vi "PatternMatch_Setting_UI.vi"(0 "Vision_Image In":T4(plugin-control), 1 "Coord?":bool, 3 "Type":string, 5 "List ROI Ref":refnum<vi>, 7 "AlgIn":T2, 9 "ProjectName":string="CDF", 11 "error in (no error)":errorcluster, 12 "ParameterIn":string, 14 "RootPath":path) -> (6 "ParameerOut":string, 10 "Cancel?":bool, 15 "error out":errorcluster)   [LabVIEW 2019]
uses:
  Controls/Parttern Match/Analysis_PatternMatch_Result.ctl
  Controls/V_Analysis_Type.ctl
  Controls/_UI Command Cluster/Pattern Match_UI Command.ctl
  <vilib>/Utility/miscctls.llb/LVPointTypeDef.ctl
  Controls/Analysis_Setting.ctl
  Controls/Parttern Match/Analysis_PatternMatch_Parameter.ctl
  <vilib>/vision/Image Controls.llb/IMAQ Image.ctl
  11e1650d-9a27-4c98-b785-94bb4e51b252.vi
  fe4c8c9f-3b30-4d10-b5c7-71603a67618a.vi
  c6f29bbc-09ff-4359-9596-1a03bc10ebeb.vi
  a50e33b9-da3b-4096-9a32-63f0ae2ad806.vi
  7765c890-54c4-40a3-a063-9b2138e01ba1.vi
  ff688e6c-f413-41b3-9d93-3794729c7324.vi
  <vilib>/JDP Science/JSONtext/JSON text to Variant.vi
  <vilib>/JDP Science/JSONtext/Variant to JSON Text.vi
  <vilib>/vision/NI_Vision_Development_Module.lvlib
  <vilib>/userdefined/High Color/IMAQdx.ctl
panel:
  out "ListROI":T1
  out "Algout":T2=enum."G_PatternMatching"
  out "Matches (real-world)":T3(array[cluster]) {"Bounding Box"."y" format="%.2f"; "Bounding Box"."x" format="%.2f"; "Score" format="%.2f"; "Scale" format="%.2f"; "Angle" format="%.2f"; "Position"."y" format="%.2f"; "Position"."x" format="%.2f"}
  in  "SetROI":bool
  out "ROI":T1
  out "Template Image":T4(plugin-control)
  in  "Cancel":bool
  in  "Done":bool
  in  "PatternMatchTab":T5(tab)
  in  "Y Position Offset":i32
  in  "X Position Offset":i32
  in  "Match Parameters":T6={"Number of Matches Requested"=1, "Minimum Match Score"=750.0, "Angle Ranges"=[]} {"Angle Ranges"."End Angle" min=-360 max=360; "Angle Ranges"."Start Angle" min=-360 max=360; "Minimum Match Score" min=0 max=1000; "Number of Matches Requested" min=1 max=9999}
  in  "Algorithm":i32(ring)=1 items=["All", "Low Discrepancy Sampling", "Grayscale Value Pyramid", "Gradients Pyramid"]
  in  "Advanced Options":cluster{"Item":u16, "Value":dbl}[](array[cluster])=[{"Item"=1, "Value"=1.0}, {"Item"=103, "Value"=1.0}] {"Item" items=["LD Sampling - Minimum Constrast"=0, "LD Sampling - Enable Subpixel Accuracy"=1, "LD Sampling - Search Strategy"=2, "LD Sampling - Subpixel Iterations"=3, "LD Sampling - Subpixel Tolerance"=4, "LD Sampling - Initial Match List Length"=5, "LD Sampling - Match List Reduction Factor"=6, "LD Sampling - Initial Step Size"=7, "LD Sampling - Intermediate Angular Accuracy"=8, "-"=9, "Pyramid - Max Pyramid Level"=100, "Pyramid - Minimum Contrast"=102, "Pyramid - Enable Subpixel Accuracy"=103, "Pyramid - Subpixel Iterations"=104, "Pyramid - Subpixel Tolerance"=105, "Pyramid - Initial Match List Length"=106, "Pyramid - Match List Reduction Factor"=107, "Pyramid - Intermediate Angular Accuracy"=108, "Pyramid - Process Border Matches"=109, "Pyramid - Min Match Separation Distance"=111, "Pyramid - Min Match Separation Angle"=112, "Pyramid - Max Match Overlap"=113, "Pyramid - Max Cache in MB"=114, "Pyramid - Clear Cache"=115]}
  out "Matches":T7[](array[typedef]) {"Bounding Box"."y" format="%.2f"; "Bounding Box"."x" format="%.2f"; "Score" format="%.2f"; "Scale" format="%.2g"; "Angle" format="%.2f"; "Position"."y" format="%.2f"; "Position"."x" format="%.2f"}
  in  "Vision_Image":T4(plugin-control)
  in  "Run Algorithm":bool
  in  "SetTemplate":bool
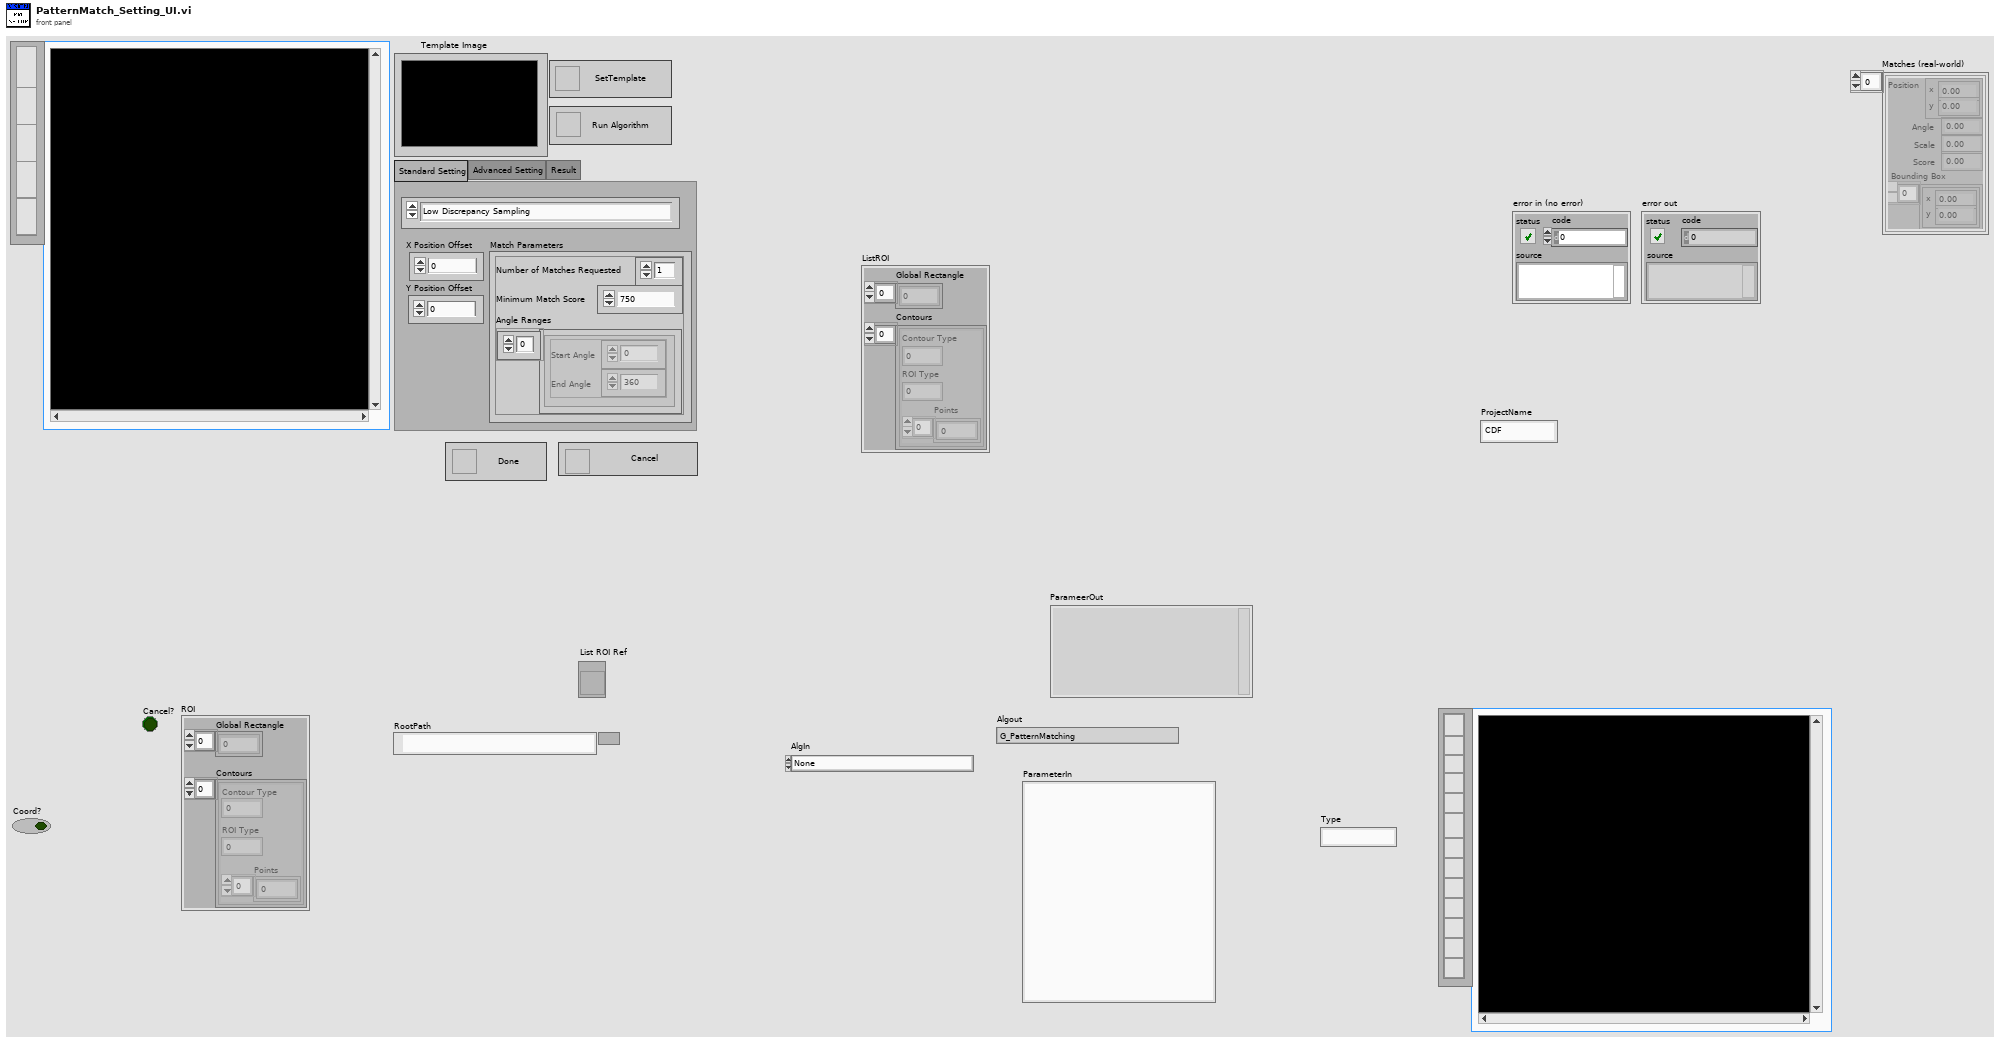
[diagram p1: front panel]
types:
  T1 = cluster{"Global Rectangle":i32[], "Contours":cluster{"Contour Type":u32, "ROI Type":u32, "Points":i32[]}[]}
  T2 = typedef "V_Analysis_Type.ctl" = enum16{"None", "C_Color Pattern Matching", "G_PatternMatching", "G_ShapeDectect", "G_GeometricMatch", "B_Area Check"}
  T3 = cluster{"Position":cluster{"x":sgl, "y":sgl}, "Angle":sgl, "Scale":sgl, "Score":sgl, "Bounding Box":cluster{"x":sgl, "y":sgl}[]}[]
  T4 = typedef "IMAQ Image.ctl" = refnum<image>
  T5 = enum32{"Standard Setting", "Advanced Setting", "Result"}
  T6 = cluster{"Number of Matches Requested":i32, "Minimum Match Score":sgl, "Angle Ranges":cluster{"Start Angle":sgl, "End Angle":sgl}[]}
  T7 = typedef "Analysis_PatternMatch_Result.ctl" = cluster{"Position":cluster{"x":sgl, "y":sgl}, "Angle":sgl, "Scale":sgl, "Score":sgl, "Bounding Box":cluster{"x":sgl, "y":sgl}[]}
  T8 = typedef "Image Type" = u32
  T9 = typedef "Pattern Match_UI Command.ctl" = enum16{"Init", "Done", "Cancel", "RunAlgorithm", "SetTemplate", "SetROI", "ClearOverlay", "Load Template", "Draw Overlay", "Offset", "Draw Curve"}
  T10 = typedef "LVPointTypeDef.ctl" = cluster{"Horizontal":i16, "Vertical":i16}
  T11 = typedef "IMAQdx.ctl" = refnum<k21>
  T12 = typedef "Analysis_Setting.ctl" = cluster{"PreProcess":T2, "Parameter":string}
  T13 = enum8{"Enabled", "Disabled", "Disabled and Grayed Out"}
  T14 = typedef "ROI Descriptor" = cluster{"Global Rectangle":i32[], "Contours":cluster{"ID":enum32{"External", "Internal"}, "Type":u32, "Coordinates":i32[]}[]}
  T15 = cluster{"Algorithm":i32, "Match Parameters":cluster{"Number of Matches Requested":i32, "Minimum Match Score":sgl, "Angle Ranges":cluster{"Start Angle":sgl, "End Angle":sgl}[]}, "ROI Descriptor":T14, "Advanced Options":cluster{"Item":u16, "Value":dbl}[], "Template path":string}
  T16 = typedef "Analysis_PatternMatch_Parameter.ctl" = cluster{"Algorithm":i32, "Match Parameters":cluster{"Number of Matches Requested":i32, "Minimum Match Score":sgl, "Angle Ranges":cluster{"Start Angle":sgl, "End Angle":sgl}[]}, "ROI Descriptor":T14, "Advanced Options":cluster{"Item":u16, "Value":dbl}[], "Template path":string, "XOffset":i32, "YOffset":i32}
  T17 = cluster{"Algorithm":i32, "Match Parameters":cluster{"Number of Matches Requested":i32, "Minimum Match Score":sgl, "Angle Ranges":cluster{"Start Angle":sgl, "End Angle":sgl}[]}, "ROI":cluster{"Global Rectangle":i32[], "Contours":cluster{"Contour Type":u32, "ROI Type":u32, "Points":i32[]}[]}, "Advanced Options":cluster{"Item":u16, "Value":dbl}[], string, i32, i32}
  T18 = cluster{"Contour Type":u32, "ROI Type":u32, "Points":i32[]}[]
  T19 = enum16{"Init", "Done", "Cancel", "RunAlgorithm", "SetTemplate", "SetROI", "ClearOverlay"}
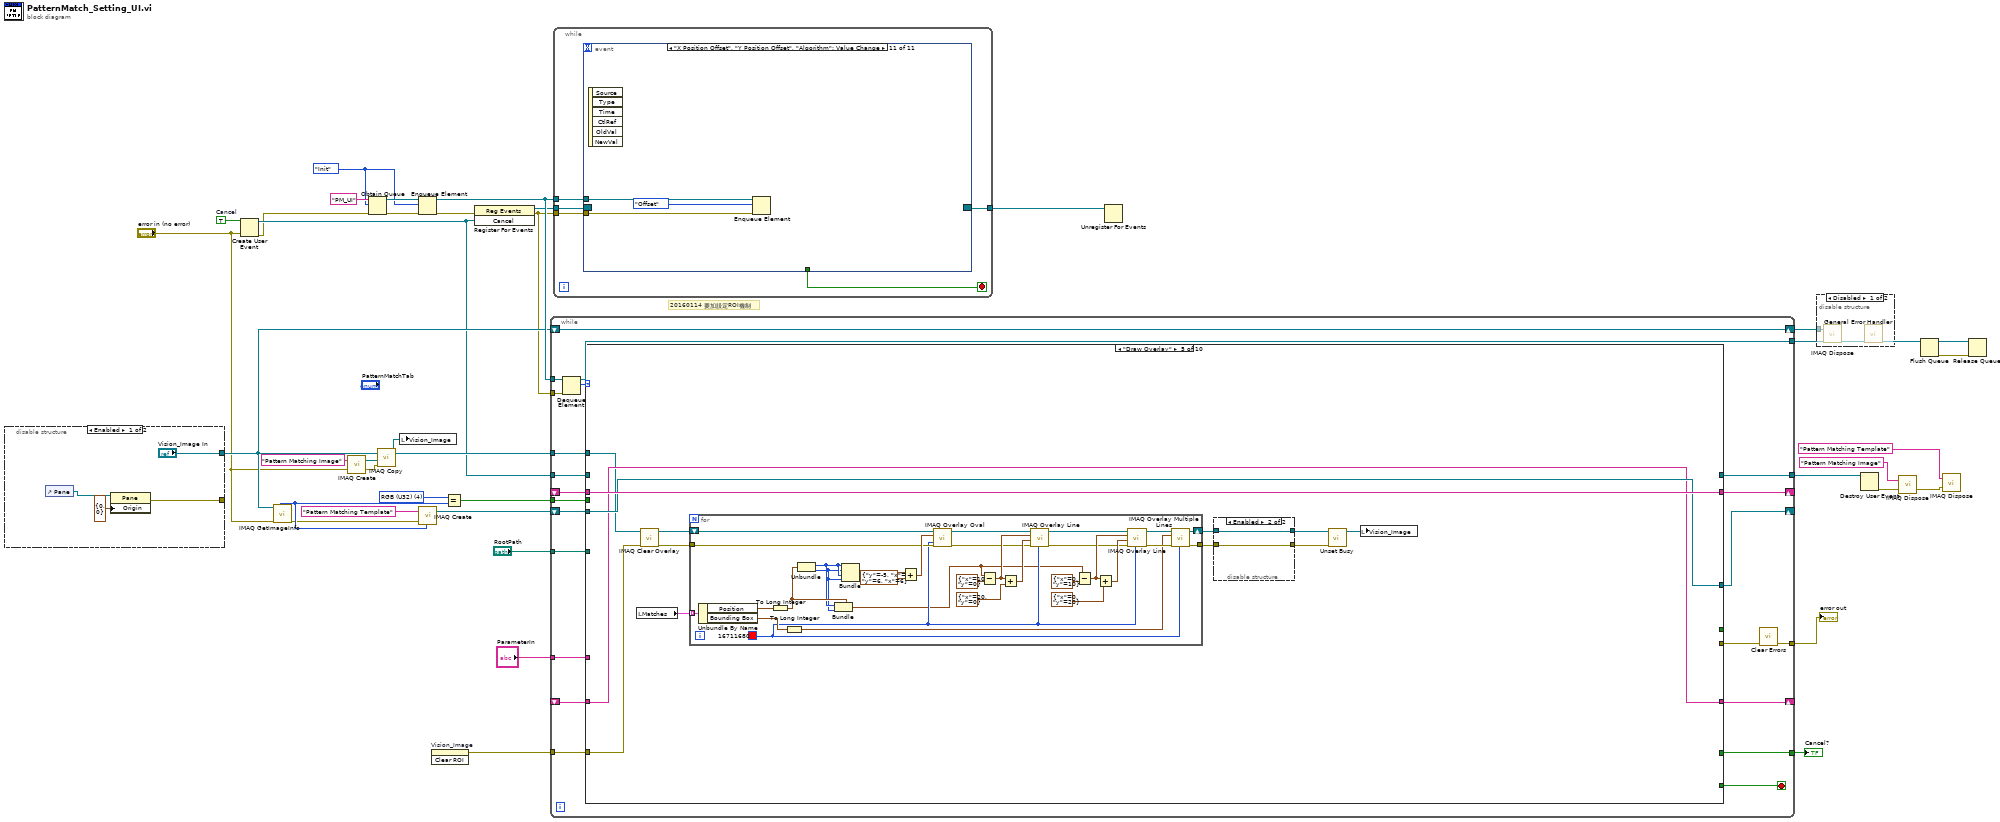
[diagram p0: block diagram]
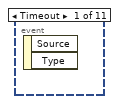
[diagram p2: hidden frame]
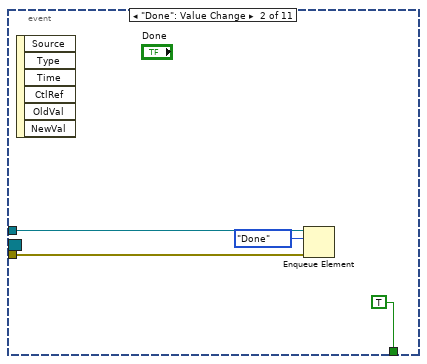
[diagram p3: hidden frame]
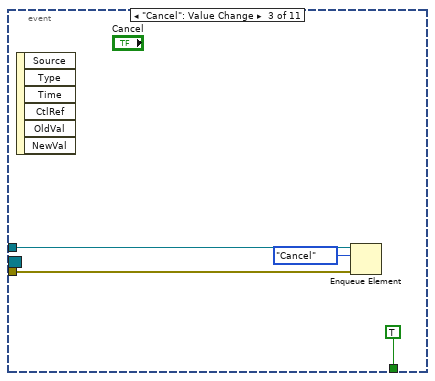
[diagram p4: hidden frame]
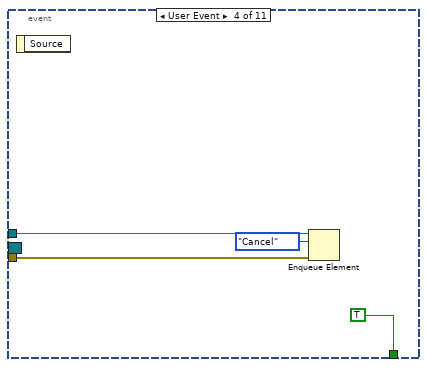
[diagram p5: hidden frame]
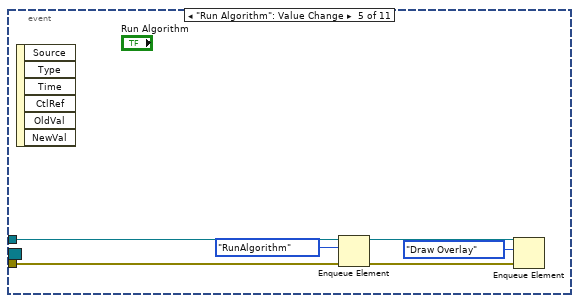
[diagram p6: hidden frame]
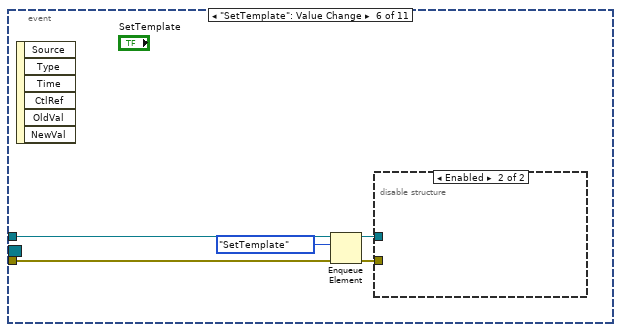
[diagram p7: hidden frame]
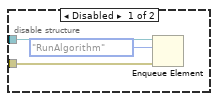
[diagram p8: hidden frame]
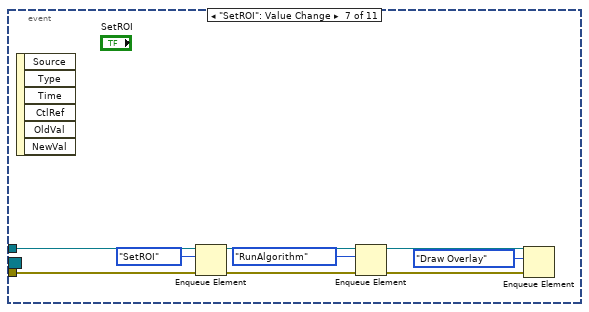
[diagram p9: hidden frame]
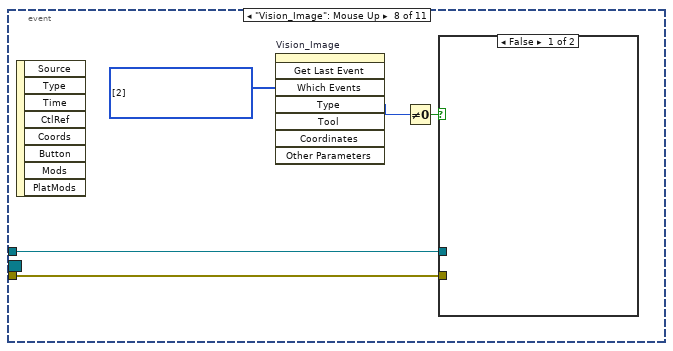
[diagram p10: hidden frame]
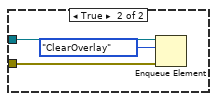
[diagram p11: hidden frame]
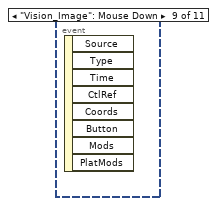
[diagram p12: hidden frame]
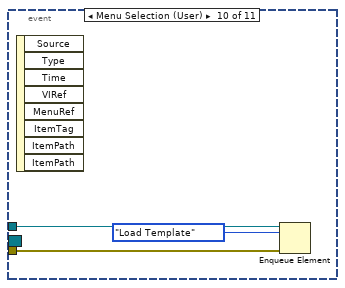
[diagram p13: hidden frame]
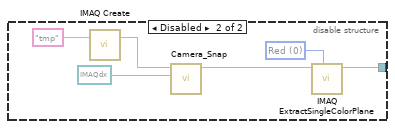
[diagram p14: hidden frame]
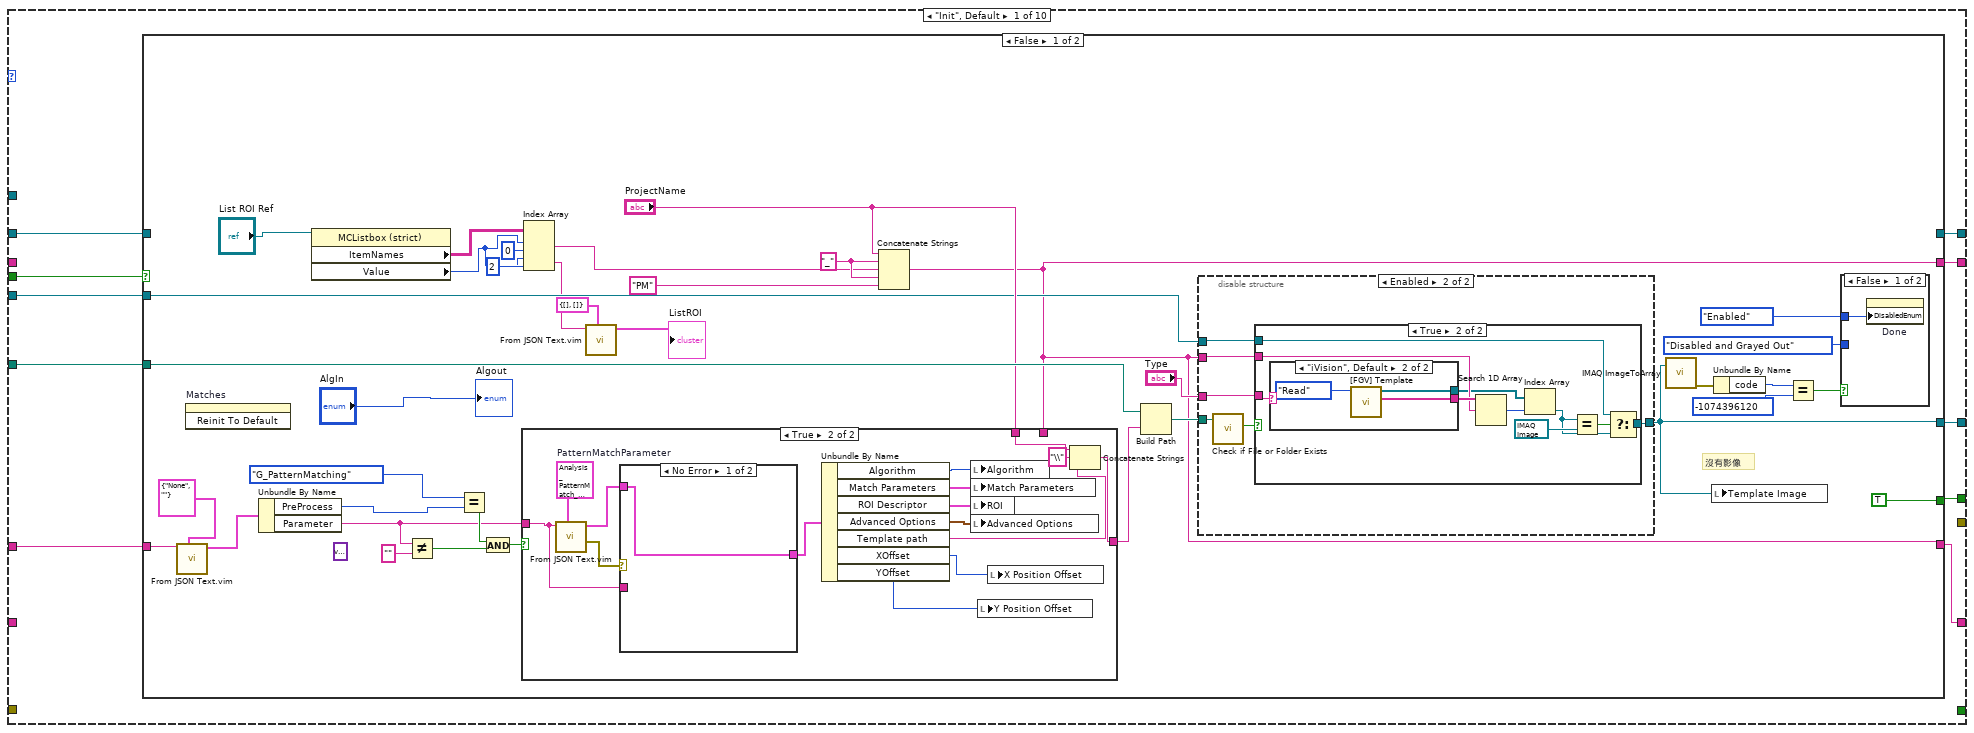
[diagram p16: hidden frame]
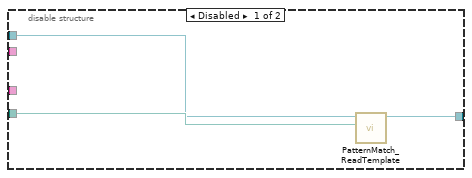
[diagram p17: hidden frame]
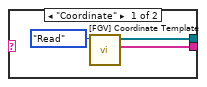
[diagram p19: hidden frame]
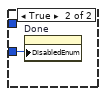
[diagram p20: hidden frame]
diagram:
  w18 = TRUE  # Cancel
  w20 = T8 4 items=["Grayscale (U8)", "Grayscale (I16)", "Grayscale (SGL)", "Complex (CSG)", "RGB (U32)", "HSL (U32)", "RGB (U64)", "Grayscale (U16)"] ("x")
  w19 = Pattern_Match_UI_Command."Init"
  # "20160114 要加設定ROI機制"
  n1 = disable-structure shown="Enabled" {
    disable-tunnel: ["Vision_Image In" w44] -> w24
    disable-tunnel: [w39 _] -> _
    frame Enabled {
      n2 = control-ref of="Pane"() -> (w41:refnum<vi>)
      n3 = property class="Pane"(reference=w41, "Origin"=T10 {"Horizontal"=0, "Vertical"=0}) -> (error out=w39:errorcluster)  [unwired: 1 in, 1 out]
    }
    frame Disabled {
      w43 = 0 items=["Red", "Green", "Blue", "Hue", "Saturation", "Luminance", "Value", "Intensity"] ("Color Plane")
      n4 = call "IMAQ Create"("Image Name"="tmp") -> ("New Image"=w46:T4)  [unwired: 4 in, 1 out]
      n5 = call "Camera_Snap.vi"("Camera Session In"=T11 refnum, "Image In"=w46) -> ("New Image"=w45:T4)  [unwired: 8 in, 1 out]
      n6 = call "IMAQ ExtractSingleColorPlane"("Color Plane"=w43, "Image Src"=w45) -> ("Image Dst Out"=w44:T4)  [unwired: 2 in, 7 out]
    }
  }
  n7 = Create User Event(user event datatype=w18, error in="error in (no error)") -> (user event=w15:refnum<user-event>, error out=w6:errorcluster)
  n8 = call "IMAQ GetImageInfo"("error in (no error)"="error in (no error)", "Image"=w24) -> ("error out"=w4:errorcluster, "Image Type"=w21:T8)  [unwired: 2 in, 6 out]
  n9 = call "IMAQ Create"("Image Name"="Pattern Matching Image", "error in (no error)"="error in (no error)") -> ("New Image"=w33:T4, "error out"=w5:errorcluster)  [unwired: 3 in]
  n10 = Obtain Queue(name (unnamed)="PM_UI", element data type=w19, error in (no error)=w6) -> (queue out=w30:refnum<queue>, error out=w29:errorcluster)  [unwired: 2 in, 1 out]
  n11 = call "IMAQ Copy"("error in (no error)"=w5, "Image Dst"=w33, "Image Src"=w24) -> ("Image Dst Out"=w32:T4)  [unwired: 3 in, 1 out]
  n12 = local write "Vision_Image"(w32) -> ()
  n13 = Enqueue Element(queue=w30, element=w19, error in (no error)=w29) -> (queue out=w26:refnum<queue>, error out=w12:errorcluster)  [unwired: 1 in, 1 out]
  n14 = call "IMAQ Create"("Image Name"="Pattern Matching Template", "Image Type"=w21, "error in (no error)"=w4) -> ("New Image"=w23:T4)  [unwired: 2 in, 1 out]
  n15 = invoke on="Vision_Image" class="ImageControl" method="Clear ROI"() -> (error out=w35:errorcluster)  [unwired: 3 in, 2 out]
  n16 = Equal?(x=w20, y=w21) -> (x = y?=w16:bool)
  n17 = register-events(error in=w12, w15) -> (reference out=w17:refnum<event-registration>, error out=w11:errorcluster)  [unwired: 1 in]
  n18 = while {
    shift-right: [w70] -> w38
    shift-left: w24 -> [w70]
    tunnel: [w66] -> w37
    tunnel: w35 -> [w52]
    tunnel: w32 -> [w69]
    tunnel: w26 -> [w64]
    tunnel: w11 -> [w62]
    tunnel: [w61] -> w25
    shift-right: [w60] -> _
    shift-left: _ -> [w59]
    shift-right: [w57] -> _
    shift-left: w23 -> [w68]
    shift-right: [w58] -> _
    shift-left: _ -> [w67]
    tunnel: "RootPath" -> [w56]
    tunnel: w16 -> [w55]
    tunnel: w15 -> [w54]
    tunnel: [w53] -> w14
    tunnel: [w51] -> w2
    tunnel: "ParameterIn" -> [w49]
    stop <- w65 stop-if-true
    n19 = Dequeue Element(queue=w64, error in (no error)=w62) -> (queue out=w61:refnum<queue>, element=w63:T9)  [unwired: 1 in, 2 out]
    n20 = case shown="\"Draw Overlay\"" w63 {
      tunnel: [_ TRUE w211 _ _ _ _ _ _ _] -> w65
      tunnel: w69 -> [_ w196 w210 _ w267 _ _ _ _ _]
      tunnel: w68 -> [w75 _ w209 w215 w269 w317 w395 w405 w419 w446]
      tunnel: [_ _ w211 _ _ _ _ _ _ _] -> w66
      tunnel: w67 -> [_ w193 w207 w213 w268 w318 w396 w406 w420 w430]
      tunnel: [w79 w195 w208 w220 w270 w319 w397 w407 w421 _] -> w60
      tunnel: w59 -> [_ w195 w208 w220 w270 w319 w397 w407 w421 _]
      tunnel: [w77 w193 w207 w213 w268 w318 w396 w406 w420 w430] -> w58
      tunnel: [w80 T4 refnum ("Template Out") T4 refnum ("Template Out") w215 w269 w314 w395 w405 w411 w432] -> w57
      tunnel: [w78 FALSE _ _ _ w316 _ _ _ _] -> _
      tunnel: w56 -> [w76 _ _ _ _ w315 _ _ w418 w431]
      tunnel: w55 -> [w74 _ _ _ _ _ _ _ _ _]
      tunnel: w54 -> [w73 w191 w205 _ _ _ _ _ _ _]
      tunnel: [w72 w191 w205 _ _ _ _ _ _ _] -> w53
      tunnel: w52 -> [_ _ _ _ w264 _ _ _ _ _]
      tunnel: [_ _ _ w212 _ _ _ _ _ _] -> w50
      tunnel: w49 -> [w71 _ _ _ _ _ _ _ _ _]
      frame "Init", Default {
        n21 = case shown="False" w74 {
          tunnel: [w105 _] -> w80
          tunnel: [w82 _] -> w79
          tunnel: [TRUE _] -> w78
          tunnel: [w82 _] -> w77
          tunnel: w76 -> [w116 _]
          tunnel: w75 -> [w106 _]
          tunnel: w73 -> [_ w182]
          tunnel: [_ w180] -> w72
          tunnel: w71 -> [w84 _]
          frame False {
            (unwired) variant
            w113 = "_" ("string")
            # "沒有影像"
            n22 = call "From JSON Text.vim"("Data Type and Default Value"=T12 {"PreProcess"=enum."None", "Parameter"=""} ("Analysis_Setting In"), "JSON"=w84) -> ("Data out"=w85:T12)  [unwired: 8 in, 1 out]
            n23 = invoke on="Matches" class="Arr (strict)" method="Reinit To Default"() -> ()  [unwired: 3 in, 3 out]
            n24 = Unbundle By Name(w85) -> ("PreProcess"=w83:T2, "Parameter"=w108:string)
            n25 = property class="MCListbox (strict)"(reference="List ROI Ref") -> ("ItemNames"=w92:string[][], "Value"=w91:i32)  [unwired: 1 in, 2 out]
            n26 = Not Equal?(x=w108, y="") -> (x != y?=w111:bool)
            n27 = Equal?(x=V_Analysis_Type."G_PatternMatching", y=w83) -> (x = y?=w112:bool)
            n28 = And(x=w112, y=w111) -> (x .and. y?=w109:bool)
            n29 = Index Array(array=w92, index (row) #1=w91, index (col) #1=0 ("disabled index (col)"), index (row) #2=w91, index (col) #2=2 ("disabled index (col)")) -> (element #1=w90:string, element #2=w88:string)
            n30 = call "From JSON Text.vim"("Data Type and Default Value"=T1 {"Global Rectangle"=[], "Contours"=[]} ("ROI"), "JSON"=w88) -> ("Data out"=→"ListROI":T1)  [unwired: 8 in, 1 out]
            n31 = Concatenate Strings("ProjectName", w113, w90, w113, "PM" ("string")) -> (w82:string)
            n32 = case shown="True" w109 {
              tunnel: [w146 w153] -> w81
              tunnel: "ProjectName" -> [w147 w156]
              tunnel: w108 -> [_ w159]
              tunnel: w82 -> [w148 _]
              frame False {
                n33 = invoke on="Y Position Offset" class="DigNum (strict)" method="Reinit To Default"() -> ()  [unwired: 3 in, 3 out]
                n34 = invoke on="X Position Offset" class="DigNum (strict)" method="Reinit To Default"() -> ()  [unwired: 3 in, 3 out]
                n35 = invoke on="Algorithm" class="Ring (strict)" method="Reinit To Default"() -> ()  [unwired: 3 in, 3 out]
                n36 = case shown="True" "Coord?" {
                  frame False {
                    n37 = invoke on="Match Parameters" class="Clust (strict)" method="Reinit To Default"() -> ()  [unwired: 3 in, 3 out]
                  }
                  frame True {
                    n38 = local write "Match Parameters"(T6 {"Number of Matches Requested"=1, "Minimum Match Score"=750.0, "Angle Ranges"=[{"Start Angle"=0.0, "End Angle"=360.0}]} ("Match Parameters")) -> ()
                  }
                }
                n39 = invoke on="Advanced Options" class="Arr (strict)" method="Reinit To Default"() -> ()  [unwired: 3 in, 3 out]
                n40 = Concatenate Strings(w147, "\\" ("string"), w148) -> (w146:string)
                "ROI" <- T1 {"Global Rectangle"=[], "Contours"=[]} ("ROI")
              }
              frame True {
                w167 = T16 {"Algorithm"=2, "Match Parameters"={"Number of Matches Requested"=1, "Minimum Match Score"=750.0, "Angle Ranges"=[]}, "ROI Descriptor"={"Global Rectangle"=[], "Contours"=[]}, "Advanced Options"=[{"Item"=1, "Value"=1.0}, {"Item"=103, "Value"=1.0}], "Template path"="", "XOffset"=0, "YOffset"=0}  # PatternMatchParameter
                n41 = call "From JSON Text.vim"("Data Type and Default Value"=w167, "JSON"=w159) -> ("error out"=w160:errorcluster, "Data out"=w158:T16)  [unwired: 8 in]
                n42 = case shown="No Error" w160 {
                  tunnel: w159 -> [_ w179]
                  tunnel: [w168 w177] -> w157
                  tunnel: w158 -> [w168 w178]
                  frame No Error {
                  }
                  frame Error {
                    w170 = 0 ("XOffset")
                    n43 = call "From JSON Text.vim"("Data Type and Default Value"=T15 {"Algorithm"=2, "Match Parameters"={"Number of Matches Requested"=1, "Minimum Match Score"=750.0, "Angle Ranges"=[]}, "ROI Descriptor"={"Global Rectangle"=[], "Contours"=[]}, "Advanced Options"=[{"Item"=1, "Value"=1.0}, {"Item"=103, "Value"=1.0}], "Template path"=""} ("PatternMatchParameter"), "JSON"=w179) -> ("Data out"=w176:T15)  [unwired: 8 in, 1 out]
                    n44 = Unbundle(w176) -> ("Algorithm"=w175:i32, "Match Parameters"=w174:T6, "ROI Descriptor"=w173:T14, "Advanced Options"=w172:cluster{"Item":u16, "Value":dbl}[], "Template path"=w171:string)
                    n45 = Bundle(cluster=w178, "Algorithm"=w175, "Match Parameters"=w174, "ROI Descriptor"=w173, "Advanced Options"=w172, "Template path"=w171, "XOffset"=w170, "YOffset"=w170) -> (w177:T16)
                  }
                }
                n46 = Unbundle By Name(w157) -> ("Algorithm"=w166:i32, "Match Parameters"=w165:T6, "ROI Descriptor"=w164:T14, "Advanced Options"=w163:cluster{"Item":u16, "Value":dbl}[], "Template path"=w154:string, "XOffset"=w162:i32, "YOffset"=w161:i32)
                n47 = local write "Algorithm"(w166) -> ()
                n48 = local write "Match Parameters"(w165) -> ()
                n49 = local write "ROI"(w164) -> ()
                n50 = local write "Advanced Options"(w163) -> ()
                n51 = local write "Y Position Offset"(w161) -> ()
                n52 = local write "X Position Offset"(w162) -> ()
                n53 = Concatenate Strings(w156, "\\" ("string"), w154) -> (w153:string)
              }
            }
            n54 = Build Path(base path=w116, name or relative path=w81) -> (appended path=w107:path)
            n55 = disable-structure shown="Enabled" {
              disable-tunnel: w107 -> [w120 w125]
              disable-tunnel: w106 -> [w119 w122]
              disable-tunnel: [w118 w123] -> w105
              disable-tunnel: w82 -> [_ w126]
              disable-tunnel: "Type" -> [_ w121]
              frame Disabled {
                n56 = call "PatternMatch_ReadTemplate.vi"("template path"=w120, "Template"=w119) -> ("Template Out"=w118:T4)  [unwired: 8 in, 1 out]
              }
              frame Enabled {
                n57 = call <vilib>:"Check if File or Folder Exists.vi"("path"=w125) -> ("file or folder exists?"=w124:bool)  [unwired: 8 in, 2 out]
                n58 = case shown="True" w124 {
                  tunnel: w126 -> [_ w136]
                  tunnel: [w127 w128] -> w123
                  tunnel: w122 -> [w127 w130]
                  tunnel: w121 -> [_ w133]
                  frame False {
                  }
                  frame True {
                    n59 = case shown="\"iVision\", Default" w133 {
                      tunnel: [w139 w142] -> w137
                      tunnel: [w140 w141] -> w134
                      frame "Coordinate" {
                        n60 = call "[FGV] Coordinate Template.vi"("Command"=enum16{"Initialize", "Save", "Read"}."Read") -> ("Image Name Array"=w139:string[], "Image Array"=w140:T4[])  [unwired: 8 in, 1 out]
                      }
                      frame "iVision", Default {
                        n61 = call "[FGV] Template.vi"("Command"=enum16{"Initialize", "Save", "Read"}."Read") -> ("Image Name Array"=w142:string[], "Image Array"=w141:T4[])  [unwired: 8 in, 1 out]
                      }
                    }
                    n62 = Search 1D Array(1D array=w137, element=w136) -> (index of element=w135:i32)  [unwired: 1 in]
                    n63 = Index Array(array=w134, index=w135) -> (element=w129:T4)
                    n64 = Equal?(x=w129, y=T4 refnum) -> (x = y?=w131:bool)
                    n65 = Select(t=w130, s=w131, f=w129) -> (s? t:f=w128:T4)
                  }
                }
              }
            }
            n66 = call "IMAQ ImageToArray"("Image"=w105) -> ("error out"=w102:errorcluster)  [unwired: 3 in, 4 out]
            n67 = local write "Template Image"(w105) -> ()
            n68 = Unbundle By Name(w102) -> ("code"=w101:i32)
            n69 = Equal?(x=w101, y=-1074396120) -> (x = y?=w99:bool)
            n70 = case shown="False" w99 {
              tunnel: T13."Disabled and Grayed Out" ("Disabled") -> [_ w145]
              tunnel: T13."Enabled" ("Disabled") -> [w144 _]
              frame False {
                n71 = property on="Done" class="Bool"("DisabledEnum"=w144) -> ()  [unwired: 2 in, 2 out]
              }
              frame True {
                n72 = property on="Done" class="Bool"("DisabledEnum"=w145) -> ()  [unwired: 2 in, 2 out]
              }
            }
            "Algout" <- "AlgIn"
          }
          frame True {
            # "輸入進來若是RGB則關閉"
            n73 = One Button Dialog(message="The Input Image Error,Image RGB", button name ("OK")="Cancel") -> (true=w181:bool)
            n74 = Generate User Event(user event=w182, event data cluster=w181) -> (user event out=w180:refnum<user-event>)  [unwired: 2 in, 1 out]
          }
        }
      }
      frame "Done" {
        w200 = T12 {"PreProcess"=enum."None", "Parameter"=""}  # Analysis_Setting
        w197 = T16 {"Algorithm"=2, "Match Parameters"={"Number of Matches Requested"=1, "Minimum Match Score"=750.0, "Angle Ranges"=[]}, "ROI Descriptor"={"Global Rectangle"=[], "Contours"=[]}, "Advanced Options"=[{"Item"=1, "Value"=1.0}, {"Item"=103, "Value"=1.0}], "Template path"="", "XOffset"=0, "YOffset"=0}  # PatternMatchParameter
        n75 = call "Imaq Dispose"("Image"=w196) -> ()  [unwired: 5 in, 1 out]
        n76 = local read "Match Parameters"() -> (w199:T6)
        n77 = local read "Algorithm"() -> (w198:i32)
        n78 = local read "Advanced Options"() -> (w202:cluster{"Item":u16, "Value":dbl}[])
        n79 = local read "Y Position Offset"() -> (w189:i32)
        n80 = local read "X Position Offset"() -> (w190:i32)
        n81 = local read "ROI"() -> (w203:T1)
        n82 = Bundle By Name(cluster=w197, "Algorithm"=w198, "Match Parameters"=w199, "ROI Descriptor"=w203, "Advanced Options"=w202, "Template path"=w193, "XOffset"=w190, "YOffset"=w189) -> (w188:T16)
        n83 = call "To JSON Text.vim"("Anything"=w188) -> ("<JSON>"=w187:string)  [unwired: 9 in, 1 out]
        n84 = Bundle By Name(cluster=w200, "PreProcess"=V_Analysis_Type."G_PatternMatching" ("Analysis"), "Parameter"=w187) -> (w186:T12)
        n85 = call "To JSON Text.vim"("Anything"=w186) -> ("<JSON>"=→"ParameerOut":string)  [unwired: 9 in, 1 out]
      }
      frame "Cancel" {
        w211 = TRUE
        n86 = call "Imaq Dispose"("Image"=w209) -> ()  [unwired: 5 in, 1 out]
        n87 = call "Imaq Dispose"("Image"=w210) -> ()  [unwired: 5 in, 1 out]
      }
      frame "RunAlgorithm" {
        n88 = call "IMAQ GetImageInfo"("Image"=w215) -> ("Y Resolution"=w219:i32, "X Resolution"=w218:i32)  [unwired: 3 in, 6 out]
        n89 = Equal To 0?(x=w218) -> (x = 0?=w217:bool)
        n90 = Equal To 0?(x=w219) -> (x = 0?=w216:bool)
        n91 = Or(x=w217, y=w216) -> (x .or. y?=w214:bool)
        n92 = case shown="False" w214 {
          tunnel: w215 -> [w224 _]
          tunnel: w213 -> [w223 _]
          tunnel: [w222 _] -> w212
          frame False {
            # "Jesse\nPattern match takes too long.\nOnly need to learn template one time"
            n93 = invoke on="Vision_Image" class="ImageControl" method="Clear ROI"() -> (error out=w234:errorcluster)  [unwired: 3 in, 2 out]
            n94 = local read "Vision_Image"() -> (w226:T4)
            n95 = call <vilib>:"Set Busy.vi"("error in (no error)"=w234) -> ("error out"=w233:errorcluster)  [unwired: 9 in, 1 out]
            n96 = local read "ListROI"() -> (w221:T1)
            n97 = local read "ROI"() -> (w225:T1)
            n98 = call "IMAQ Clear Overlay"("error in (no error)"=w233, "Image"=w226) -> ("error out"=w227:errorcluster, "Image Out"=w231:T4)  [unwired: 8 in]
            n99 = disable-structure shown="Enabled" {
              disable-tunnel: w224 -> [w244 _]
              disable-tunnel: w227 -> [w243 w252]
              disable-tunnel: "Match Parameters" -> [w241 w257]
              disable-tunnel: "Algorithm" -> [w240 w258]
              disable-tunnel: "Advanced Options" -> [w239 w254]
              disable-tunnel: w231 -> [w238 w255]
              disable-tunnel: [w237 w259] -> w232
              disable-tunnel: w225 -> [w235 w253]
              disable-tunnel: w223 -> [_ w251]
              disable-tunnel: [_ w249] -> w222
              disable-tunnel: w221 -> [_ _]
              frame Disabled {
                w246 = 0 items=["All", "Low Discrepancy Sampling", "Grayscale Value Pyramid", "Gradients Pyramid"] ("Algorithm")
                n100 = call "IMAQ Learn Pattern 4"("Algorithm"=w246, "error in (no error)"=w243, "Angle Range"=cluster{"Start Angle":sgl, "End Angle":sgl} {"Start Angle"=0.0, "End Angle"=360.0}, "Image"=w244) -> ("error out"=w242:errorcluster, "Template Image Out"=w236:T4)  [unwired: 5 in, 1 out]
                n101 = call "IMAQ Match Pattern 4"("Image"=w238, "Algorithm"=w240, "Template Image"=w236, "ROI Descriptor"=w235, "Parameters"=w241, "error in (no error)"=w242, "Advanced Options"=w239) -> ("Matches (pixel)"=w237:T3)  [unwired: 4 in, 4 out]
              }
              frame Enabled {
                w248 = 0
                n102 = Bundle("Algorithm"=w258, "Match Parameters"=w257, "ROI"=w253, "Advanced Options"=w254, w251, w248, w248) -> (w256:T17)  [unwired: 1 in]
                n103 = call "PatternMatch_MainFunction.vi"("PatternMatchParameter"=w256, "Vision_Image In"=w255, "ROI Descriptor"=T14 {"Global Rectangle"=[], "Contours"=[]}, "error in"=w252) -> ("Matches"=w259:T7[], "Matches (real-world)"=→"Matches (real-world)":T3, "error out"=w249:errorcluster)  [unwired: 7 in, 2 out]
              }
            }
            "Matches" <- w232
          }
          frame True {
            n104 = One Button Dialog(message="No Template is Set~!!!\nPlease Set Template Before Analyze~!!") -> ()  [unwired: 1 in, 1 out]
          }
        }
      }
      frame "Draw Overlay" {
        n105 = local read "Matches"() -> (w272:T7[])
        n106 = call "IMAQ Clear Overlay"("error in (no error)"=w264, "Image"=w267) -> ("error out"=w265:errorcluster, "Image Out"=w266:T4)  [unwired: 8 in]
        n107 = for {
          tunnel: w272 -> [w291] mode=indexing
          tunnel: w265 -> [w287]
          shift-right: [w285] -> w271
          shift-left: w266 -> [w290]
          tunnel: [w284] -> w262
          w286 = u32 16711680 ("Color")
          n108 = Unbundle By Name(w291) -> ("Position"=w289:cluster{"x":sgl, "y":sgl}, "Bounding Box"=w288:cluster{"x":sgl, "y":sgl}[])
          n109 = To Long Integer(number=w289) -> (32bit integer=w283:cluster{"x":i32, "y":i32})
          n110 = To Long Integer(number=w288) -> (32bit integer=w292:cluster{"x":i32, "y":i32}[])
          n111 = Unbundle(w283) -> ("x"=w281:i32, "y"=w280:i32)
          n112 = Bundle(cluster=w283, "x"=w281, "y"=w280) -> (w282:cluster{"x":i32, "y":i32})
          n113 = Bundle("x"=w281, "y"=w280, "x"=w281, "y"=w280) -> (w307:cluster{"x":i32, "y":i32, "x":i32, "y":i32})  [unwired: 1 out]
          n114 = Add(x=w307, y=cluster{"y":i32, "x":i32, "y":i32, "x":i32} {"y"=-5, "x"=-5, "y"=6, "x"=6}) -> (x+y=w305:cluster{i32, i32, i32, i32})
          n115 = call "IMAQ Overlay Oval"("Color"=w286, "error in (no error)"=w287, "Bounding Rectangle"=w305, "Image"=w290) -> ("error out"=w295:errorcluster, "Image Out"=w309:T4)  [unwired: 2 in, 4 out]
          n116 = Subtract(x=w282, y=cluster{"x":i32, "y":i32} {"x"=10, "y"=0}) -> (x-y=w303:cluster{"x":i32, "y":i32})
          n117 = Add(x=w303, y=cluster{"x":i32, "y":i32} {"x"=20, "y"=0}) -> (x+y=w301:cluster{"x":i32, "y":i32})
          n118 = call "IMAQ Overlay Line"("Color"=w286, "error in (no error)"=w295, "End Point"=w301, "Start Point"=w303, "Image"=w309) -> ("error out"=w294:errorcluster, "Image Out"=w296:T4)  [unwired: 1 in, 4 out]
          n119 = Subtract(x=w282, y=cluster{"x":i32, "y":i32} {"x"=0, "y"=10}) -> (x-y=w299:cluster{"x":i32, "y":i32})
          n120 = Add(x=w299, y=cluster{"x":i32, "y":i32} {"x"=0, "y"=20}) -> (x+y=w300:cluster{"x":i32, "y":i32})
          n121 = call "IMAQ Overlay Line"("Color"=w286, "error in (no error)"=w294, "End Point"=w300, "Start Point"=w299, "Image"=w296) -> ("error out"=w293:errorcluster, "Image Out"=w308:T4)  [unwired: 1 in, 4 out]
          n122 = call "IMAQ Overlay Multiple Lines"("Color"=w286, "error in (no error)"=w293, "Line End Points"=w292, "Image"=w308) -> ("error out"=w284:errorcluster, "Image Out"=w285:T4)  [unwired: 2 in, 4 out]
        }
        n123 = disable-structure shown="Enabled" {
          disable-tunnel: w271 -> [w277 w279]
          disable-tunnel: [w276 w279] -> w263
          disable-tunnel: w262 -> [w275 w278]
          disable-tunnel: [w274 w278] -> w261
          frame Disabled {
            n124 = local read "ListROI"() -> (w273:T1)
            n125 = call "IMAQ Overlay ROI"("error in (no error)"=w275, "ROI Descriptor"=w273, "Image"=w277) -> ("error out"=w274:errorcluster, "Image Out"=w276:T4)  [unwired: 7 in]
          }
          frame Enabled {
          }
        }
        n126 = call <vilib>:"Unset Busy.vi"("error in (no error)"=w261) -> ()  [unwired: 10 in, 1 out]
        n127 = local write "Vision_Image"(w263) -> ()
      }
      frame "SetTemplate" {
        # "沒有影像"
        # "-1074396120"
        n128 = call "IMAQ GetImageInfo"("Image"=w317) -> ("error out"=w313:errorcluster)  [unwired: 3 in, 7 out]
        n129 = Unbundle By Name(w313) -> ("code"=w312:i32)
        n130 = Equal?(x=w312, y=-1074396120) -> (x = y?=w310:bool)
        n131 = case shown="False" w310 {
          tunnel: [w322 TRUE] -> w320
          frame False {
            n132 = Two Button Dialog(message="Template Already Exist, You Sure to Create New Template?") -> (T button?=w322:bool)  [unwired: 2 in]
          }
          frame True {
          }
        }
        n133 = case shown="True" w320 {
          tunnel: w317 -> [w324 w332]
          tunnel: w318 -> [_ w331]
          tunnel: [_ w330] -> w316
          tunnel: w315 -> [_ w329]
          tunnel: [w324 w328] -> w314
          frame False {
          }
          frame True {
            n134 = local read "Algorithm"() -> (w327:i32)
            n135 = property on="Vision_Image" class="ImageControl"() -> ("ROI"=w337:T1)  [unwired: 2 in, 2 out]
            n136 = Unbundle By Name(w337) -> ("Contours"=w336:T18, "Global Rectangle"=w333:i32[])
            n137 = case shown="3" w327 {
              tunnel: [w338 w339 w340 w341] -> w326
              frame 0 {
                w338 = 0 items=["All", "Low Discrepancy Sampling", "Grayscale Value Pyramid", "Gradients Pyramid"] ("Algorithm")
              }
              frame 1, Default {
                w339 = 1 items=["All", "Low Discrepancy Sampling", "Grayscale Value Pyramid", "Gradients Pyramid"] ("Algorithm")
              }
              frame 2 {
                w340 = 2 items=["All", "Low Discrepancy Sampling", "Grayscale Value Pyramid", "Gradients Pyramid"] ("Algorithm")
              }
              frame 3 {
                w341 = 3 items=["All", "Low Discrepancy Sampling", "Grayscale Value Pyramid", "Gradients Pyramid"] ("Algorithm")
              }
            }
            n138 = Array Size(array=w336) -> (size(s)=w335:i32)
            n139 = Not Equal To 0?(x=w335) -> (x != 0?=w334:bool)
            n140 = case shown="True" w334 {
              tunnel: w333 -> [_ w380]
              tunnel: w332 -> [w342 w379]
              tunnel: w331 -> [_ w349]
              tunnel: [_ TRUE] -> w330
              tunnel: w329 -> [_ w345]
              tunnel: [w342 w370] -> w328
              tunnel: w326 -> [_ w364]
              tunnel: cluster{"Item":u16, "Value":dbl}[] [{"Item"=10, "Value"=0.0}, {"Item"=11, "Value"=0.0}] ("Advanced Options") -> [_ w359]
              frame False {
                n141 = One Button Dialog(message="Please Select Template On the Image") -> ()  [unwired: 1 in, 1 out]
              }
              frame True {
                n142 = local read "ProjectName"() -> (w344:string)
                n143 = local read "X Position Offset"() -> (w361:i32)
                n144 = local read "Y Position Offset"() -> (w360:i32)
                n145 = Index Array(array=w359) -> (element #1=w363:cluster{"Item":u16, "Value":dbl}, element #2=w362:cluster{"Item":u16, "Value":dbl})  [unwired: 2 in]
                n146 = call <vilib>:"Set Busy.vi"() -> ("error out"=w367:errorcluster)  [unwired: 10 in, 1 out]
                n147 = Build Path(base path=w345, name or relative path=w344) -> (appended path=w346:path)
                n148 = Bundle By Name(cluster=w363, "Value"=w361) -> (w358:cluster{"Item":u16, "Value":dbl})
                n149 = Bundle By Name(cluster=w362, "Value"=w360) -> (w357:cluster{"Item":u16, "Value":dbl})
                n150 = call "[FGV] Template.vi"("Command"=enum16{"Initialize", "Save", "Read"}."Read") -> ("Image Name Array"=w350:string[])  [unwired: 8 in, 2 out]
                n151 = call "IMAQ Extract"("Optional Rectangle"=w380, "error in (no error)"=w367, "Image Dst"=w379, "Image Src"="Vision_Image") -> ("error out"=w374:errorcluster, "Image Dst Out"=w369:T4)  [unwired: 6 in]
                n152 = Build Path(base path=w346, name or relative path=w349) -> (appended path=w376:path)
                n153 = Replace Array Subset(array=w359, new element #1=w358, new element #2=w357) -> (w356:cluster{"Item":u16, "Value":dbl}[])  [unwired: 2 in]
                n154 = Search 1D Array(1D array=w350, element=w349) -> (index of element=w351:i32)  [unwired: 1 in]
                n155 = Less Than 0?(x=w351) -> (x < 0?=w348:bool)
                n156 = call "IMAQ Learn Pattern 4"("Advanced Options"=w356, "Algorithm"=w364, "error in (no error)"=w374, "Angle Range"=cluster{"Start Angle":sgl, "End Angle":sgl} {"Start Angle"=0.0, "End Angle"=360.0}, "Image"=w369) -> ("error out"=w366:errorcluster, "Template Image Out"=w347:T4)  [unwired: 4 in, 1 out]
                n157 = case shown="True" w348 {
                  tunnel: w350 -> [_ w383]
                  tunnel: w349 -> [_ w382]
                  frame False {
                  }
                  frame True {
                    n158 = Build Array (concatenate)(w383, w382) -> (w381:string[])
                    n159 = call "[FGV] Template.vi"("Image Name Array"=w381, "Image Array"=w381, "Command"=enum16{"Initialize", "Save", "Read"}."Save") -> ()  [unwired: 6 in, 3 out]
                  }
                }
                n160 = invoke on="Vision_Image" class="ImageControl" method="Clear ROI"(error in=w374) -> ()  [unwired: 2 in, 3 out]
                n161 = Unbundle By Name(w366) -> ("code"=w373:i32)
                n162 = call "IMAQ Create"("Image Name"=w349) -> ("New Image"=w354:T4, "error out"=w355:errorcluster)  [unwired: 4 in]
                n163 = call "IMAQ Copy"("error in (no error)"=w355, "Image Dst"=w354, "Image Src"=w347) -> ("Image Dst Out"=w353:T4)  [unwired: 3 in, 1 out]
                n164 = Equal?(x=w373, y=-1074395252) -> (x = y?=w371:bool)
                n165 = case shown="False" w371 {
                  tunnel: w376 -> [w389 _]
                  tunnel: w347 -> [w388 w392]
                  tunnel: [w385 w392] -> w370
                  tunnel: w353 -> [w385 _]
                  tunnel: [w385 T4 refnum ("Image Dst Out")] -> w368
                  tunnel: w366 -> [w386 w390]
                  tunnel: [w386 w390] -> w365
                  frame False {
                    n166 = call-poly "IMAQ Write File 2"("File Path"=w389, "Image"=w388) -> ()  [unwired: 8 in, 2 out]
                    n167 = property on="Done" class="Bool"("DisabledEnum"=T13."Enabled" ("Disabled")) -> ()  [unwired: 2 in, 2 out]
                  }
                  frame True {
                    n168 = One Button Dialog(message="Invalid learn setup data.\nplease Reset Set", button name ("OK")="OK") -> ()  [unwired: 1 out]
                  }
                }
                "Template Image" <- w368
                n169 = call <vilib>:"Unset Busy.vi"("error in (no error)"=w365) -> ()  [unwired: 10 in, 1 out]
              }
            }
          }
        }
      }
      frame "SetROI" {
        n170 = property on="Vision_Image" class="ImageControl"() -> ("ROI"=w398:T1)  [unwired: 2 in, 2 out]
        n171 = Unbundle By Name(w398) -> ("Global Rectangle"=w400:i32[])
        n172 = Array Size(array=w400) -> (size(s)=w401:i32)
        n173 = Not Equal To 0?(x=w401) -> (x != 0?=w399:bool)
        n174 = case shown="True" w399 {
          tunnel: w398 -> [_ w403]
          frame False {
            n175 = One Button Dialog(message="Please Select An Area As ROI") -> ()  [unwired: 1 in, 1 out]
          }
          frame True {
            n176 = disable-structure shown="Enabled" {
              disable-tunnel: w403 -> [w404 _]
              frame Enabled {
                n177 = local write "ROI"(w404) -> ()
              }
              frame Disabled {
              }
            }
          }
        }
      }
      frame "ClearOverlay" {
        n178 = local read "Vision_Image"() -> (w409:T4)
        n179 = call "IMAQ Clear Overlay"("Image"=w409) -> ("Image Out"=w408:T4)  [unwired: 9 in, 1 out]
        n180 = local write "Vision_Image"(w408) -> ()
      }
      frame "Load Template" {
        # "這個不需要改，因為這是開放給使用者自己去選的"
        # "後面不需要去做Learn Pattern的動作，因為讀進的Pattern都是已經Learn過"
        n181 = Build Path(base path=w418, name or relative path="\\Data") -> (appended path=w417:path)
        n182 = call "File Dialog"("start path"=w417) -> ("selected path"=w416:path, "cancelled"=w415:bool, "error out"=w414:errorcluster)  [unwired: 11 in, 1 out]
        n183 = call <vilib>:"Clear Errors.vi"("error in (no error)"=w414) -> ()  [unwired: 5 in, 2 out]
        n184 = case shown="False" w415 {
          tunnel: w419 -> [w425 w426]
          tunnel: [w424 w426] -> w411
          tunnel: w416 -> [w423 _]
          frame False {
            n185 = call "PatternMatch_ReadTemplate.vi"("template path"=w423, "Template"=w425) -> ("Template Out"=w424:T4)  [unwired: 8 in, 1 out]
          }
          frame True {
          }
        }
        n186 = local write "Template Image"(w411) -> ()
        n187 = call "IMAQ ImageToArray"("Image"=w411) -> ("Image Pixels (U8)"=w412:u8[][])  [unwired: 3 in, 4 out]
        n188 = Empty Array?(array=w412) -> (empty?=w410:bool)
        n189 = case shown="False" w410 {
          frame False {
            n190 = property on="Done" class="Bool"("DisabledEnum"=T13."Enabled" ("Disabled")) -> ()  [unwired: 2 in, 2 out]
          }
          frame True {
          }
        }
      }
      frame "Offset" {
        n191 = local read "Algorithm"() -> (w445:i32)
        n192 = local read "ProjectName"() -> (w428:string)
        n193 = Build Path(base path=w431, name or relative path=w428) -> (appended path=w429:path)
        n194 = case shown="3" w445 {
          tunnel: [w461 w463 w465 w467] -> w444
          tunnel: [cluster{"Item":u16, "Value":dbl}[] [] ("Advanced Options") cluster{"Item":u16, "Value":dbl}[] [{"Item"=10, "Value"=0.0}, {"Item"=11, "Value"=0.0}] ("Advanced Options") cluster{"Item":u16, "Value":dbl}[] [{"Item"=102, "Value"=0.0}, {"Item"=103, "Value"=0.0}] ("Advanced Options") cluster{"Item":u16, "Value":dbl}[] [{"Item"=102, "Value"=0.0}, {"Item"=103, "Value"=0.0}] ("Advanced Options")] -> w427
          frame 0 {
            w461 = 0 items=["All", "Low Discrepancy Sampling", "Grayscale Value Pyramid", "Gradients Pyramid"] ("Algorithm")
          }
          frame 1, Default {
            w463 = 1 items=["All", "Low Discrepancy Sampling", "Grayscale Value Pyramid", "Gradients Pyramid"] ("Algorithm")
          }
          frame 2 {
            w465 = 2 items=["All", "Low Discrepancy Sampling", "Grayscale Value Pyramid", "Gradients Pyramid"] ("Algorithm")
          }
          frame 3 {
            w467 = 3 items=["All", "Low Discrepancy Sampling", "Grayscale Value Pyramid", "Gradients Pyramid"] ("Algorithm")
          }
        }
        n195 = Build Path(base path=w429, name or relative path=w430) -> (appended path=w435:path)
        n196 = Index Array(array=w427) -> (element #1=w450:cluster{"Item":u16, "Value":dbl}, element #2=w449:cluster{"Item":u16, "Value":dbl})  [unwired: 2 in]
        n197 = Bundle By Name(cluster=w450, "Value"="X Position Offset") -> (w448:cluster{"Item":u16, "Value":dbl})
        n198 = Bundle By Name(cluster=w449, "Value"="Y Position Offset") -> (w447:cluster{"Item":u16, "Value":dbl})
        n199 = call <vilib>:"Set Busy.vi"() -> ("error out"=w436:errorcluster)  [unwired: 10 in, 1 out]
        n200 = Replace Array Subset(array=w427, new element #1=w448, new element #2=w447) -> (w451:cluster{"Item":u16, "Value":dbl}[])  [unwired: 2 in]
        n201 = call "IMAQ Learn Pattern 4"("Advanced Options"=w451, "Algorithm"=w444, "error in (no error)"=w436, "Angle Range"=cluster{"Start Angle":sgl, "End Angle":sgl} {"Start Angle"=0.0, "End Angle"=360.0}, "Image"=w446) -> ("error out"=w434:errorcluster, "Template Image Out"=w437:T4)  [unwired: 4 in, 1 out]
        n202 = Unbundle By Name(w434) -> ("code"=w439:i32)
        n203 = Equal?(x=w439, y=-1074395252) -> (x = y?=w440:bool)
        n204 = case shown="False" w440 {
          tunnel: w435 -> [w455 _]
          tunnel: w437 -> [w454 w457]
          tunnel: [w454 w457] -> w432
          tunnel: w434 -> [w452 w456]
          tunnel: [w452 w456] -> w433
          frame False {
            n205 = call-poly "IMAQ Write File 2"("File Path"=w455, "Image"=w454) -> ()  [unwired: 8 in, 2 out]
            n206 = property on="Done" class="Bool"("DisabledEnum"=T13."Enabled" ("Disabled")) -> ()  [unwired: 2 in, 2 out]
          }
          frame True {
            n207 = One Button Dialog(message="Invalid learn setup data.\nplease Reset Set", button name ("OK")="OK") -> ()  [unwired: 1 out]
          }
        }
        n208 = call <vilib>:"Unset Busy.vi"("error in (no error)"=w433) -> ()  [unwired: 10 in, 1 out]
      }
    }
    n209 = call <vilib>:"Clear Errors.vi"("error in (no error)"=w50) -> ("error out"=w51:errorcluster)  [unwired: 5 in, 1 out]
  }
  "error out" <- w2
  "Cancel?" <- w37
  n210 = while {
    tunnel: w26 -> [w471]
    tunnel: w11 -> [w470]
    tunnel: w17 -> [w469]
    tunnel: [w468] -> w13
    stop <- w472 stop-if-true
    n211 = event shown="[10] \"X Position Offset\", \"Y Position Offset\", \"Algorithm\": Value Change" {
      selector: w469 -> [_ _ _ _ _ _ _ _ _ _ _]
      dyn-events: [_ _ _ _ _ _ _ _ _ _ _] -> w468
      timeout: _ -> [_ _ _ _ _ _ _ _ _ _ _]
      tunnel: [_ TRUE TRUE TRUE _ _ _ _ _ _ _] -> w472
      tunnel: w471 -> [_ w475 w479 w483 w490 w495 w507 w509 _ w518 w521]
      tunnel: w470 -> [_ w474 w478 w482 w489 w494 w506 w508 _ w517 w520]
      event Timeout {
        n212 = event-data() -> ()  [unwired: 1 in, 2 out]
      }
      event "Done": Value Change {
        n213 = event-data() -> ()  [unwired: 1 in, 6 out]
        n214 = Enqueue Element(queue=w475, element=Pattern_Match_UI_Command."Done", error in (no error)=w474) -> ()  [unwired: 1 in, 3 out]
      }
      event "Cancel": Value Change {
        n215 = event-data() -> ()  [unwired: 1 in, 6 out]
        n216 = Enqueue Element(queue=w479, element=Pattern_Match_UI_Command."Cancel", error in (no error)=w478) -> ()  [unwired: 1 in, 3 out]
      }
      event User Event {
        n217 = event-data() -> ()  [unwired: 1 in, 1 out]
        n218 = Enqueue Element(queue=w483, element=Pattern_Match_UI_Command."Cancel", error in (no error)=w482) -> ()  [unwired: 1 in, 3 out]
      }
      event "Run Algorithm": Value Change {
        n219 = event-data() -> ()  [unwired: 1 in, 6 out]
        n220 = Enqueue Element(queue=w490, element=Pattern_Match_UI_Command."RunAlgorithm", error in (no error)=w489) -> (queue out=w486:refnum<queue>, error out=w487:errorcluster)  [unwired: 1 in, 1 out]
        n221 = Enqueue Element(queue=w486, element=Pattern_Match_UI_Command."Draw Overlay", error in (no error)=w487) -> ()  [unwired: 1 in, 3 out]
      }
      event "SetTemplate": Value Change {
        n222 = event-data() -> ()  [unwired: 1 in, 6 out]
        n223 = Enqueue Element(queue=w495, element=Pattern_Match_UI_Command."SetTemplate", error in (no error)=w494) -> (queue out=w492:refnum<queue>, error out=w491:errorcluster)  [unwired: 1 in, 1 out]
        n224 = disable-structure shown="Enabled" {
          disable-tunnel: w492 -> [w498 _]
          disable-tunnel: w491 -> [w497 _]
          frame Disabled {
            n225 = Enqueue Element(queue=w498, element=T19."RunAlgorithm", error in (no error)=w497) -> ()  [unwired: 1 in, 3 out]
          }
          frame Enabled {
          }
        }
      }
      event "SetROI": Value Change {
        n226 = event-data() -> ()  [unwired: 1 in, 6 out]
        n227 = Enqueue Element(queue=w507, element=Pattern_Match_UI_Command."SetROI", error in (no error)=w506) -> (queue out=w504:refnum<queue>, error out=w503:errorcluster)  [unwired: 1 in, 1 out]
        n228 = Enqueue Element(queue=w504, element=Pattern_Match_UI_Command."RunAlgorithm", error in (no error)=w503) -> (queue out=w500:refnum<queue>, error out=w501:errorcluster)  [unwired: 1 in, 1 out]
        n229 = Enqueue Element(queue=w500, element=Pattern_Match_UI_Command."Draw Overlay", error in (no error)=w501) -> ()  [unwired: 1 in, 3 out]
      }
      event "Vision_Image": Mouse Up {
        w510 = i32[] [2] items=["No Event"=0, "Click Event"=1, "Draw Event"=2, "Size Event"=4, "Scroll Event"=5, "Double Click Event"=8] ("Which Events")
        n230 = event-data() -> ()  [unwired: 1 in, 8 out]
        n231 = invoke on="Vision_Image" class="ImageControl" method="Get Last Event"("Which Events"=w510) -> ("Type"=w511:i32)  [unwired: 7 in, 7 out]
        n232 = Not Equal To 0?(x=w511) -> (x != 0?=w512:bool)
        n233 = case shown="False" w512 {
          tunnel: w509 -> [_ w515]
          tunnel: w508 -> [_ w514]
          frame False {
          }
          frame True {
            n234 = Enqueue Element(queue=w515, element=Pattern_Match_UI_Command."ClearOverlay", error in (no error)=w514) -> ()  [unwired: 1 in, 3 out]
          }
        }
      }
      event "Vision_Image": Mouse Down {
        n235 = event-data() -> ()  [unwired: 1 in, 8 out]
      }
      event Menu Selection (User) {
        n236 = event-data() -> ()  [unwired: 1 in, 8 out]
        n237 = Enqueue Element(queue=w518, element=Pattern_Match_UI_Command."Load Template", error in (no error)=w517) -> ()  [unwired: 1 in, 3 out]
      }
      event "X Position Offset", "Y Position Offset", "Algorithm": Value Change {
        n238 = event-data() -> ()  [unwired: 1 in, 6 out]
        n239 = Enqueue Element(queue=w521, element=Pattern_Match_UI_Command."Offset", error in (no error)=w520) -> ()  [unwired: 1 in, 3 out]
      }
    }
  }
  n240 = Unregister For Events(event registration refnum=w13) -> ()  [unwired: 1 in, 1 out]
  n241 = disable-structure shown="Disabled" {
    disable-tunnel: w38 -> [w522 _]
    frame Disabled {
      n242 = call "IMAQ Dispose"("Image"=w522) -> ("error out"=w523:errorcluster)  [unwired: 5 in]
      n243 = call <vilib>:"General Error Handler.vi"("error in (no error)"=w523) -> ()  [unwired: 2 in, 13 out]
    }
    frame Enabled {
    }
  }
  n244 = Destroy User Event(user event=w14) -> (error out=w10:errorcluster)  [unwired: 1 in]
  n245 = call "IMAQ Dispose"("Image"="Pattern Matching Image" ("Image Name"), "error in (no error)"=w10) -> ("error out"=w8:errorcluster)  [unwired: 4 in]
  n246 = Flush Queue(queue=w25) -> (queue out=w28:refnum<queue>, error out=w27:errorcluster)  [unwired: 1 in, 1 out]
  n247 = call "IMAQ Dispose"("Image"="Pattern Matching Template" ("Image Name"), "error in (no error)"=w8) -> ()  [unwired: 4 in, 1 out]
  n248 = Release Queue(queue=w28, error in (no error)=w27) -> ()  [unwired: 1 in, 3 out]
